vi "Write TCPIP Msg Q.vi"(8 "error in (no error)":errorcluster, 10 "Actor Framework:Message Enqueuer":refnum<class "Message Enqueuer.lvclass">, 11 "subpanel (abstract) in":refnum<class "subpanel (abstract).lvclass">=refnum) -> (0 "error out":errorcluster, 3 "subpanel (abstract) out":refnum<class "subpanel (abstract).lvclass">)   [LabVIEW 2023, in "subpanel (abstract).lvclass"]
uses:
  subpanel (abstract).lvclass
  subpanel (abstract).lvclass/subpanel (abstract).ctl
  <vilib>/ActorFramework/Message Enqueuer/Message Enqueuer.lvclass
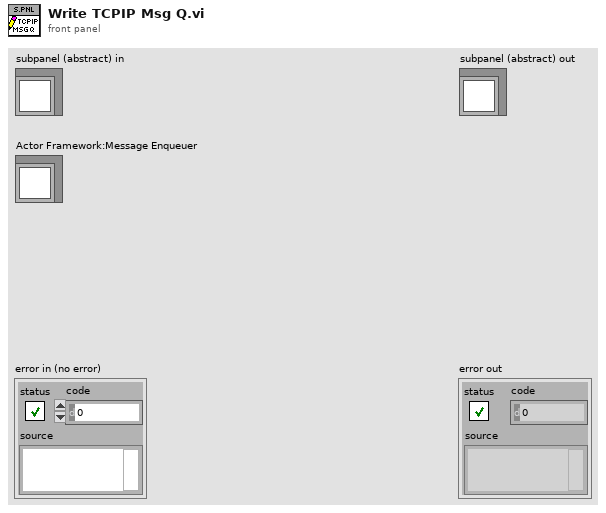
[diagram p1: front panel]
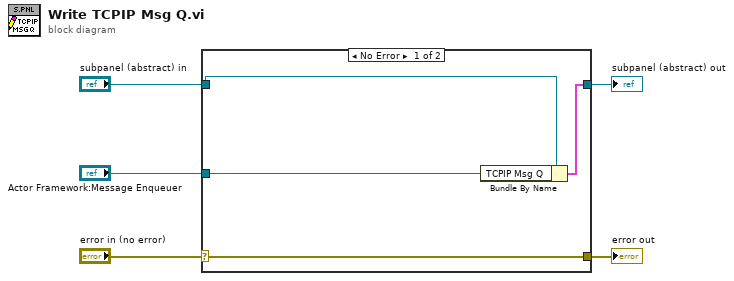
[diagram p0: block diagram]
diagram:
  n1 = case shown="No Error" "error in (no error)" {
    selector: "error in (no error)" -> [w9 w10]
    tunnel: [w9 w10] -> w4
    tunnel: [w7 w11] -> w2
    tunnel: "subpanel (abstract) in" -> [w8 w11]
    tunnel: "Actor Framework:Message Enqueuer" -> [w6 _]
    frame No Error {
      n2 = Bundle By Name(cluster=w8, "TCPIP Msg Q"=w6) -> (w7:cluster{})
    }
    frame Error {
    }
  }
  "error out" <- w4
  "subpanel (abstract) out" <- w2
